vi "Quit LabVIEW if EXE.vi"(8 "error in (no error)":errorcluster, 10 "Quit LabVIEW?":bool) -> (0 "error out":errorcluster)   [LabVIEW 2018]
doc: "Quits LabVIEW if and only if this VI is being called from inside an executable."
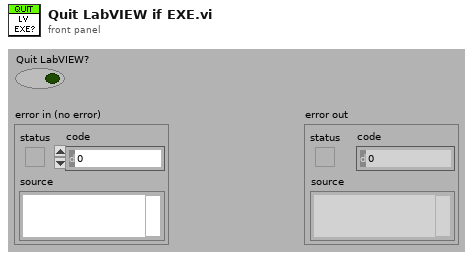
[diagram p1: front panel]
types:
  T1 = enum32{"invalid app kind", "Development System", "Run Time System", "Student Edition", "Embedded LabVIEW", "Evaluation", "Custom"}
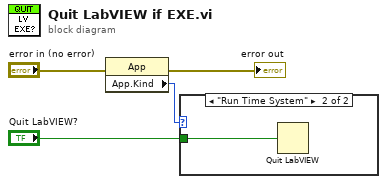
[diagram p0: block diagram]
diagram:
  n1 = property class="App"(error in="error in (no error)") -> (error out=→"error out":errorcluster, "App.Kind"=w4:T1)  [unwired: 1 in, 1 out]
  n2 = case shown="\"Run Time System\"" w4 {
    tunnel: "Quit LabVIEW?" -> [_ w5]
    frame "invalid app kind", Default {
    }
    frame "Run Time System" {
      n3 = Quit LabVIEW(quit? (T)=w5) -> ()
    }
  }
